vi "_Server Prepare Run.vi"(6 "FW Simulator":bool, 8 "error in (no error)":errorcluster, 11 "Server Method":T7 {"Expt"."Mass Range"."Res" items=["High/High", "Medium/Medium", "Low/Low", "High/Medium", "High/Low", "Medium/High", "Medium/Low", "Low/High", "Low/Medium"]}) -> (0 "error out":errorcluster, 3 "Scans":i32=5)   [LabVIEW 2015]
uses:
  Type/_Server Method.ctl
  Type/_XML Expt.ctl
  Type/_XML Lens.ctl
  Type/_Mass Range Property.ctl
  Type/_Mass Range Parameters.ctl
  Type/_RT Res Type.ctl
  Type/_RT Active Ch.ctl
  Type/_RT Parameter.ctl
  Type/_RT Expt.ctl
  Type/_Run Mode.ctl
  Type/_RT Mass Range.ctl
  Type/_RT Command.ctl
  Configuration/_Global Configuration.vi
panel:
  out "Parameter":T1 {"Expt"."Mass Range"."Resolution Type" items=["High/High", "Medium/Medium", "Low/Low", "High/Medium", "High/Low", "Medium/High", "Medium/Low", "Low/High", "Low/Medium"]}
  # "(# of Expts) X (# of Cycles)"
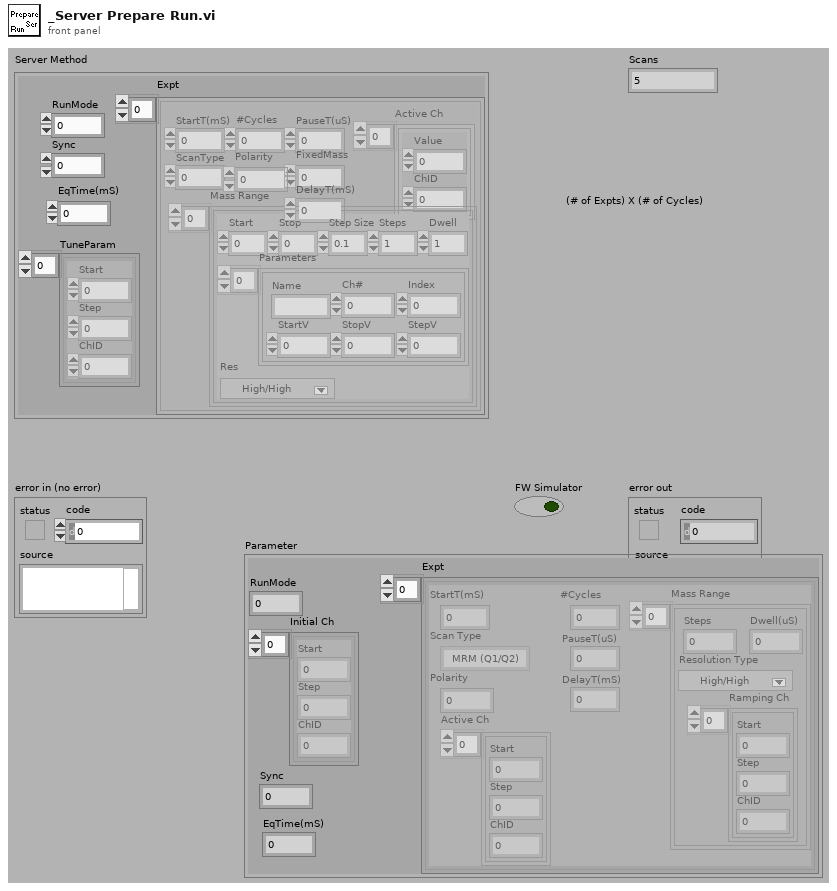
[diagram p1: front panel]
types:
  T1 = typedef "_RT Parameter.ctl" = cluster{"RunMode":i32, "Initial Ch":T2[], "Sync":u8, "Expt":T3[], "EqTime(mS)":i32}
  T2 = typedef "_RT Active Ch.ctl" = cluster{"Start":i32, "Step":i32, "ChID":i32}
  T3 = typedef "_RT Expt.ctl" = cluster{"StartT(mS)":i32, "#Cycles":i32, "Scan Type":T4, "PauseT(uS)":i32, "Polarity":u8, "DelayT(mS)":i32, "Active Ch":T2[], "Mass Range":T5[]}
  T4 = typedef "_Run Mode.ctl" = enum16{"MRM (Q1/Q2)", "Q1 Scan", "Q1 SRM", "Q2 Scan", "Q2 SRM", "Product Scan", "Precursor Scan", "Neutral Loss", "Neutral Gain"}
  T5 = typedef "_RT Mass Range.ctl" = cluster{"Steps":i32, "Dwell(uS)":i32, "Resolution Type":T6, "Ramping Ch":T2[]}
  T6 = typedef "_RT Res Type.ctl" = u16
  T7 = typedef "_Server Method.ctl" = cluster{"RunMode":i32, "Sync":u8, "Expt":T8[], "EqTime(mS)":i32, "TuneParam":T2[]}
  T8 = typedef "_XML Expt.ctl" = cluster{"StartT(mS)":i32, "#Cycles":i32, "PauseT(uS)":i32, "ScanType":i32, "Polarity":u8, "FixedMass":dbl, "DelayT(mS)":i32, "Active Ch":T9[], "Mass Range":T10[]}
  T9 = typedef "_XML Lens.ctl" = cluster{"Value":dbl, "ChID":u8}
  T10 = typedef "_Mass Range Property.ctl" = cluster{"Start":dbl, "Stop":dbl, "Step Size":dbl, "Steps":i32, "Dwell":dbl, "Parameters":T11[], "Res":T6}
  T11 = typedef "_Mass Range Parameters.ctl" = cluster{"Name":string, "Ch#":u8, "StartV":dbl, "StopV":dbl, "StepV":dbl, "Index":u8}
  T12 = typedef "_RT Configuration 2.ctl" = cluster{"Name":string, "Ch#":u8, "Min":dbl, "Max":dbl, "Def+":dbl, "Def-":dbl, "Offset":dbl, "Slope":dbl, "Type":u8, "Description":string, "SettleT":dbl}
  T13 = typedef "_RT Command.ctl" = enum16{"xml Start Run", "xml Start Actual Run", "xml Stop Run", "xml Runtime Update", "xml Get Status", "xml Get Table", "xml Set Table", "xml Get Configuration", "xml System Status", "xml Set LC Input Logic", "xml Get Data", "xml Get Info", "Start", "StartActualRun", "Stop", "Runtime Update", "Get Data", "Get Info", "Get Status", "Get Param", "Get Config", "Get Table", "Read ADC", "Set Oscillator", "Update Config", "Update Table", "Set All Pol", "Set Pol and DC", "Set Max Mass", "Toggle RP", "Toggle EL", "Set PIC", "Initialize Turbo", "Send Turbo Comm", "Close Turbo", "P1", "P2", "P3", "Send Serial", "Set LC Out", "Get LC In", "Read VAC", "Test Table", "Toggle Power", "Get Startup", "Set Startup", "Get ADC Table", "Set ADC Table", "Get Brief Status", "Get Detail Status", "Auxiliary Update", "Set CC Logics", "Set CC Input Logics", "Ignore Error", "invalid"}
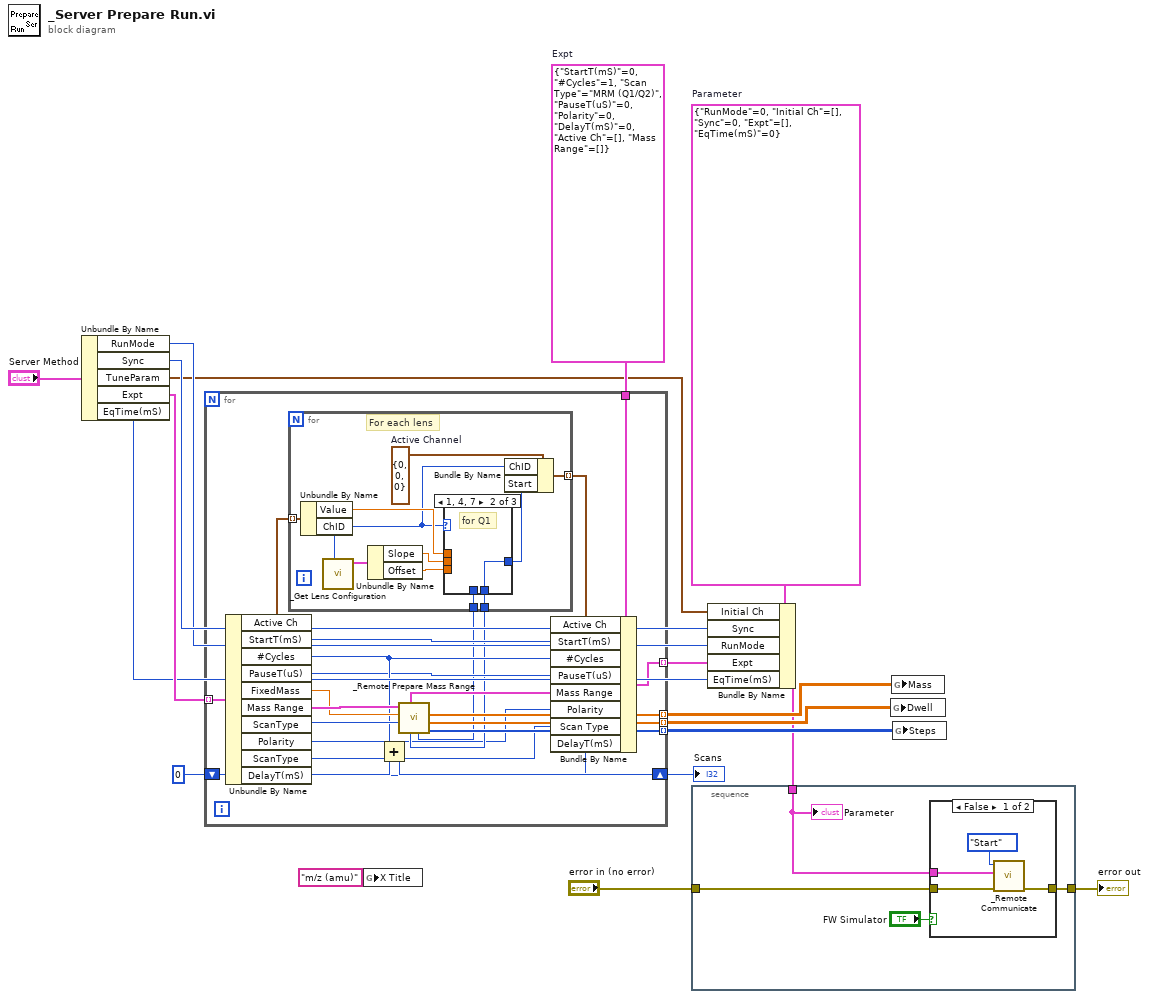
[diagram p0: block diagram]
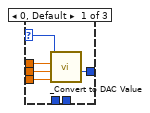
[diagram p3: hidden frame]
diagram:
  w9 = T1 {"RunMode"=0, "Initial Ch"=[], "Sync"=0, "Expt"=[], "EqTime(mS)"=0}  # Parameter
  w11 = T3 {"StartT(mS)"=0, "#Cycles"=1, "Scan Type"=enum."MRM (Q1/Q2)", "PauseT(uS)"=0, "Polarity"=0, "DelayT(mS)"=0, "Active Ch"=[], "Mass Range"=[]}  # Expt
  n1 = Unbundle By Name("Server Method") -> ("RunMode"=w4:i32, "Sync"=w5:u8, "TuneParam"=w2:T2[], "Expt"=w6:T8[], "EqTime(mS)"=w1:i32)
  n2 = for {
    tunnel: w6 -> [w40] mode=indexing
    tunnel: [w36] -> w12 mode=indexing
    tunnel: [w35] -> w13 mode=indexing
    tunnel: [w34] -> w14 mode=indexing
    shift-right: [w32] -> w15
    shift-left: 0 ("index") -> [w33]
    tunnel: w11 -> [w31]
    tunnel: [w22] -> w10 mode=indexing
    n3 = Unbundle By Name(w40) -> ("Active Ch"=w26:T9[], "StartT(mS)"=w28:i32, "#Cycles"=w29:i32, "PauseT(uS)"=w27:i32, "FixedMass"=w38:dbl, "Mass Range"=w39:T10[], "ScanType"=w37:i32, "Polarity"=w21:u8, "ScanType"=w20:i32, "DelayT(mS)"=w19:i32)
    n4 = Add(x=w29, y=w33) -> (x+y=w32:i32)
    n5 = call "_Remote Prepare Mass Range.vi"("Run Mode"=w37, "Fixed Mass (amu)"=w38, "GUI Mass Ranges"=w39) -> ("Steps"=w34:i32[], "Dwell (ms)"=w35:dbl[], "Mass"=w36:dbl[], "Init Q2 Mass"=w23:i32, "Init Q1 Mass"=w24:i32, "RT Mass Ranges"=w30:T5[])  [unwired: 3 out]
    n6 = for {
      tunnel: [w47] -> w25 mode=indexing
      tunnel: w26 -> [w46] mode=indexing
      tunnel: w24 -> [w42]
      tunnel: w23 -> [w41]
      w49 = T2 {"Start"=0, "Step"=0, "ChID"=0}  # Active Channel
      # "For each lens"
      n7 = Unbundle By Name(w46) -> ("Value"=w45:dbl, "ChID"=w44:u8)
      n8 = call "_Get Lens Configuration.vi"("Channel #"=w44) -> ("Lens Configuration"=w43:T12)  [unwired: 1 in, 5 out]
      n9 = Unbundle By Name(w43) -> ("Slope"=w51:dbl, "Offset"=w50:dbl)
      n10 = case shown="1, 4, 7" w44 {
        selector: w44 -> [w52 _ _]
        tunnel: w45 -> [w56 _ _]
        tunnel: w51 -> [w55 _ _]
        tunnel: w50 -> [w54 _ _]
        tunnel: [w53 w57 w58] -> w48
        tunnel: w42 -> [_ w57 _]
        tunnel: w41 -> [_ _ w58]
        frame 0, Default {
          n11 = call "_Convert to DAC Value.vi"("Offset"=w54, "Slop"=w55, "Number"=w56, "Channel"=w52) -> ("DAC Value"=w53:i32)  [unwired: 2 in, 5 out]
        }
        frame 1, 4, 7 {
          # "for Q1"
        }
        frame 2, 5, 9 {
          # "for Q3"
        }
      }
      n12 = Bundle By Name(cluster=w49, "ChID"=w44, "Start"=w48) -> (w47:T2)
    }
    n13 = Bundle By Name(cluster=w31, "Active Ch"=w25, "StartT(mS)"=w28, "#Cycles"=w29, "PauseT(uS)"=w27, "Mass Range"=w30, "Polarity"=w21, "Scan Type"=w20, "DelayT(mS)"=w19) -> (w22:T3)
  }
  "Scans" <- w15
  n14 = global write "_Global Configuration.vi" "X Title"("m/z (amu)" ("X Title")) -> ()
  n15 = Bundle By Name(cluster=w9, "Initial Ch"=w2, "Sync"=w5, "RunMode"=w4, "Expt"=w10, "EqTime(mS)"=w1) -> (w8:T1)
  n16 = stacked-sequence {
    tunnel: [w62] -> w17
    tunnel: w8 -> [w61]
    tunnel: "error in (no error)" -> [w60]
    frame #0 {
      n17 = case shown="False" "FW Simulator" {
        tunnel: [w65 w67] -> w62
        tunnel: w61 -> [w64 _]
        tunnel: w60 -> [w63 w67]
        frame False {
          n18 = call "_Remote Communicate.vi"("error in (no error)"=w63, "Parameter"=w64, "Command"=_RT_Command."Start") -> ("error out"=w65:errorcluster)  [unwired: 3 in, 3 out]
        }
        frame True {
        }
      }
      "Parameter" <- w61
    }
  }
  "error out" <- w17
  n19 = global write "_Global Configuration.vi" "Dwell"(w13) -> ()
  n20 = global write "_Global Configuration.vi" "Mass"(w12) -> ()
  n21 = global write "_Global Configuration.vi" "Steps"(w14) -> ()
